vi "Validate and register ROI group clicked on.vi"(9 "Coords":T1) -> (0 "error out":errorcluster, 1 "Array is not empty":bool, 3 "Index of group clicked on":i16)   [LabVIEW 2013]
uses:
  <vilib>/Utility/miscctls.llb/LVPoint32TypeDef.ctl
  Global variables/gl_Functional Imaging-Global variables.vi
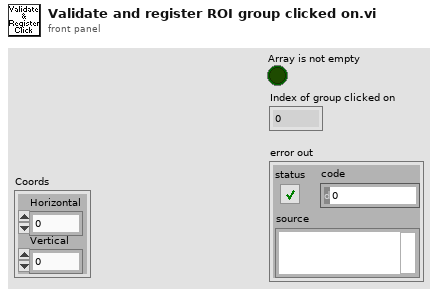
[diagram p1: front panel]
types:
  T1 = typedef "LVPoint32TypeDef.ctl" = cluster{"Horizontal":i32, "Vertical":i32}
  T2 = typedef "Functional Imging UI Refs.ctl" = cluster{"Menu ref":refnum<k9>, "Image control":refnum<vi>, "VI ref":refnum<vi>, "XGrapher":refnum<vi>, "Smoothing":refnum<vi>, "POI Averaging":refnum<vi>, "Normalize":refnum<vi>, "POI data points in each trial":refnum<vi>, "Channel":refnum<vi>, "Experiment data folder path":refnum<vi>, "[ROI vis]":refnum<vi>, "[Groups] visbl":T3, "Group Name":refnum<vi>, "POI index":refnum<vi>, "Trial No.":refnum<vi>, "Intensity Zoom":refnum<vi>, "Trial Cursor Enabled":refnum<vi>, "Number of Trials (ind 1)":refnum<vi>, "Number of Trials (ind 2)":refnum<vi>, "MiniScans Available":refnum<vi>, "POI Available":refnum<vi>, "Defer graph updates":refnum<vi>, "Waveform selector":refnum<vi>, "#of selected POI":refnum<vi>, "#of selected MiniScans":refnum<vi>, "#of selected groups":refnum<vi>, "Max Z-Projection":refnum<vi>, "Z-Plane Selector":refnum<vi>, "Index of miniscan point to visualise":refnum<vi>, "ROI vis. mode":refnum<vi>, "Total # of points":refnum<vi>, "Index of group clicked on":refnum<vi>, "Pane 1":refnum<vi>, "Pane 2":refnum<vi>, "Pane 3":refnum<vi>, "Pane 4":refnum<vi>, "Pane 5":refnum<vi>, "Pane 6":refnum<vi>, "Deselect all ROI":refnum<vi>, "Deselect all groups":refnum<vi>}
  T3 = typedef "Groups array referecne.ctl" = refnum<vi>
  T4 = typedef "Group sel cluster.ctl" = cluster{"Group number":string, "Group Name":string, "Visibility":bool, "Highlight":bool}
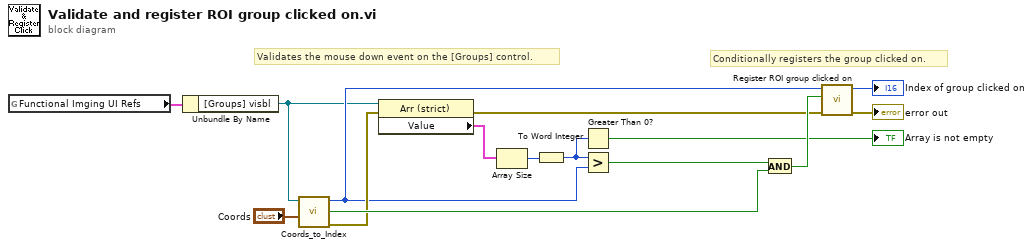
[diagram p0: block diagram]
diagram:
  # "Conditionally registers the group clicked on."
  # "Validates the mouse down event on the [Groups] control."
  n1 = global read "gl_Functional Imaging-Global variables.vi" "Functional Imging UI Refs"() -> (w2:T2)
  n2 = Unbundle By Name(w2) -> ("[Groups] visbl"=w3:T3)
  n3 = call "Coords_to_Index.vi"("coords"="Coords", "Array ref"=w3) -> ("error out"=w9:errorcluster, "row index"=w7:i16, "V In Range?"=w11:bool)  [unwired: 5 in, 2 out]
  n4 = property on="Property Node" class="Arr (strict)"(reference=w3, error in=w9) -> (error out=w8:errorcluster, "Value"=w1:T4[])  [unwired: 1 out]
  n5 = Array Size(array=w1) -> (size(s)=w13:i32)
  n6 = To Word Integer(number=w13) -> (16bit integer=w5:i16)
  n7 = Greater Than 0?(x=w5) -> (x > 0?=→"Array is not empty":bool)
  n8 = Greater?(x=w5, y=w7) -> (0:w12:bool)
  n9 = And(x=w12, y=w11) -> (x .and. y?=w10:bool)
  n10 = call "Register ROI group clicked on.vi"("error in (no error)"=w8, "Valid"=w10, "Group index"=w7) -> ("error out"=→"error out":errorcluster, "Group index"=→"Index of group clicked on":i16)  [unwired: 7 in]
